vi "Authorization Read License File.vi"(8 "error in (no error)":errorcluster, 11 "Debug?":bool) -> (0 "error out":errorcluster, 3 "Authorization":T1)   [LabVIEW 2011]
uses:
  Authorization Data.ctl
  Authorization Global.vi
  <vilib>/xml/Load XML File.vi
  <vilib>/xml/Close Reference(Node).vi
  <vilib>/xml/NI_XML.lvlib
  Program Files/National Instruments/LabVIEW 2011/resource/objmgr/DOMUserDefRef.rc
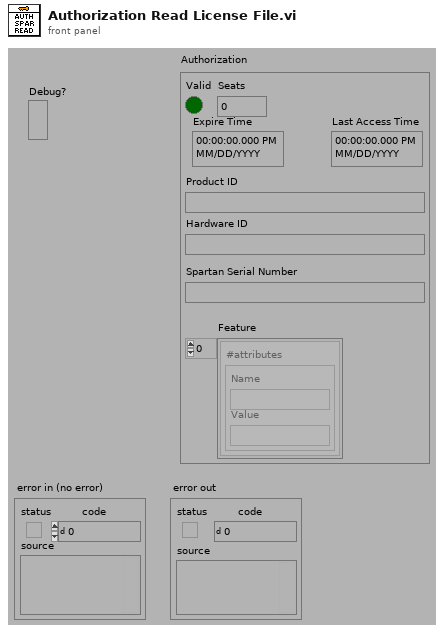
[diagram p1: front panel]
types:
  T1 = typedef "Authorization Data.ctl" = cluster{"Valid":bool, "Seats":i32, "Expire Time":timestamp, "Last Access Time":timestamp, "Product ID":string, "Hardware ID":string, "Spartan Serial Number":string, "Feature":cluster{"#attributes":cluster{"Name":string, "Value":string}}[]}
  T2 = enum32{"invalid app kind", "Development System", "Run Time System", "Student Edition", "Embedded LabVIEW", "Evaluation", "Custom"}
  T3 = cluster{"#attributes":cluster{"Name":string, "Value":string}}[]
  T4 = cluster{"#attributes":cluster{"Name":string, "Value":string}}
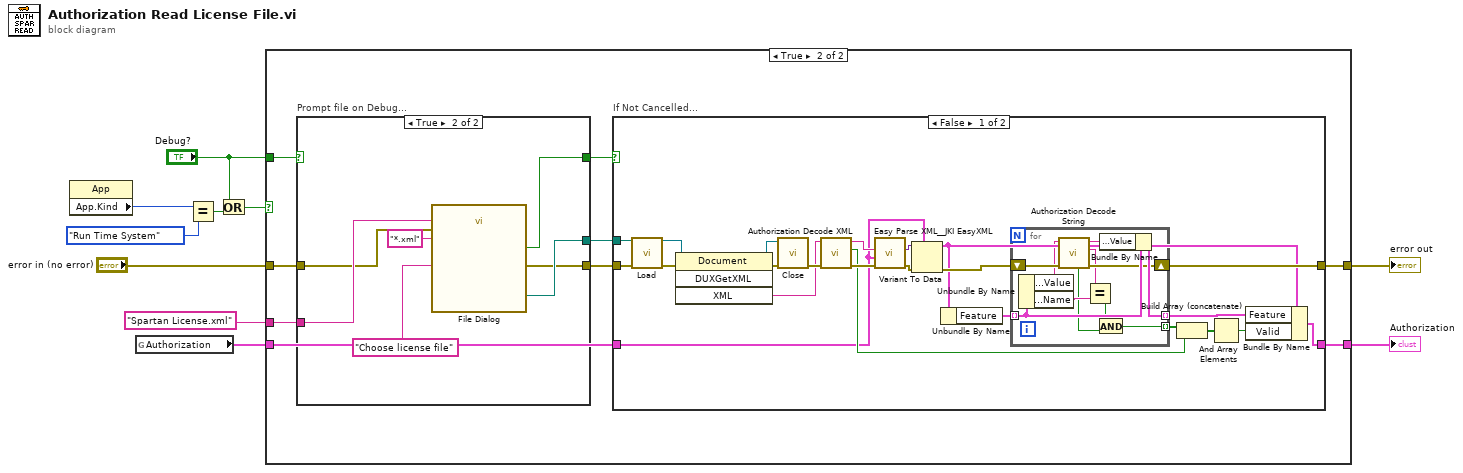
[diagram p0: block diagram]
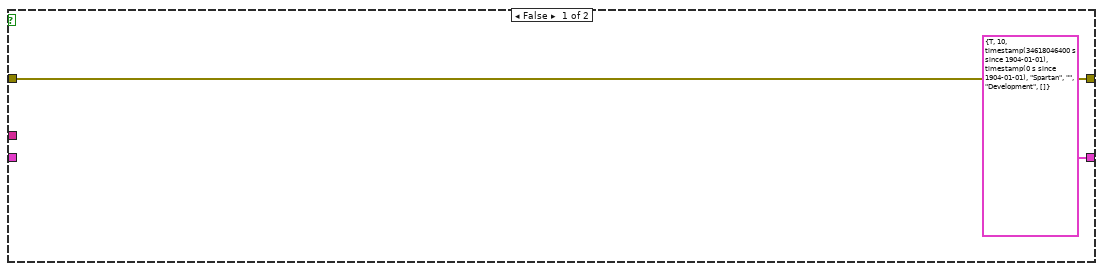
[diagram p2: hidden frame]
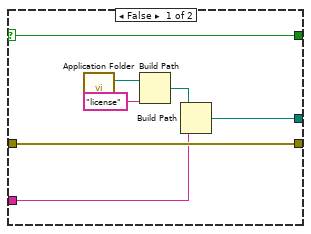
[diagram p4: hidden frame]
diagram:
  n1 = property class="App"() -> ("App.Kind"=w6:T2)  [unwired: 2 in, 2 out]
  n2 = global read "Authorization Global.vi" "Authorization"() -> (w1:T1)
  n3 = Equal?(x=w6, y=T2."Run Time System" ("t")) -> (x = y?=w4:bool)
  n4 = Or(x="Debug?", y=w4) -> (x .or. y?=w3:bool)
  n5 = case shown="True" w3 {
    tunnel: "error in (no error)" -> [w12 w16]
    tunnel: [w12 w21] -> w9
    tunnel: [T1 {"Valid"=TRUE, "Seats"=10, "Expire Time"=timestamp(34618046400 s since 1904-01-01), "Last Access Time"=timestamp(0 s since 1904-01-01), "Product ID"="Spartan", "Hardware ID"="", "Spartan Serial Number"="Development", "Feature"=[]} ("Authorization") w20] -> w8
    tunnel: "Spartan License.xml" ("default name") -> [_ w18]
    tunnel: "Debug?" -> [_ w17]
    tunnel: w1 -> [_ w13]
    frame False {
    }
    frame True {
      n6 = case "Prompt file on Debug..." shown="True" w17 {
        selector: w17 -> [w63 _]
        tunnel: [w58 w71] -> w19
        tunnel: w18 -> [w59 w68]
        tunnel: [w64 w66] -> w15
        tunnel: w16 -> [w64 w67]
        tunnel: [w63 w65] -> w14
        frame False {
          n7 = call "Application Folder.vi"() -> ("Application Folder"=w62:path)  [unwired: 3 in]
          n8 = Build Path(base path=w62, name or relative path="license" ("Relative Path (\"\" - Folder)")) -> (appended path=w60:path)
          n9 = Build Path(base path=w60, name or relative path=w59) -> (appended path=w58:path)
        }
        frame True {
          n10 = call "File Dialog"("prompt"="Choose license file", "default name"=w68, "error in"=w67, "pattern (all files)"="*.xml") -> ("selected path"=w71:path, "cancelled"=w65:bool, "error out"=w66:errorcluster)  [unwired: 8 in, 1 out]
        }
      }
      n11 = case "If Not Cancelled..." shown="False" w14 {
        tunnel: [w42 w57] -> w21
        tunnel: [w41 w56] -> w20
        tunnel: w19 -> [w40 _]
        tunnel: w15 -> [w39 w57]
        tunnel: w13 -> [w22 w56]
        frame False {
          n12 = call-poly <vilib>:"Load.vi"("path to XML document"=w40, "error in (no error)"=w39) -> ("DOM document out"=w44:refnum<k20>, "error out"=w43:errorcluster)  [unwired: 11 in, 1 out]
          n13 = invoke class="Document" method="DUXGetXML"(reference=w44, error in=w43) -> (reference out=w37:refnum<k20>, error out=w38:errorcluster, "XML"=w35:string)  [unwired: 2 in, 1 out]
          n14 = call-poly <vilib>:"Close.vi"("error in (no error)"=w38, "node"=w37) -> ("error out"=w36:errorcluster)  [unwired: 7 in]
          n15 = call "Authorization Decode XML.vi"("error in (no error)"=w36, "Encoded XML String"=w35) -> ("error out"=w32:errorcluster, "Valid"=w23:bool, "Decoded XML String"=w31:string)  [unwired: 7 in]
          n16 = call "Easy Parse XML__JKI EasyXML.vi"("error in (no error)"=w32, "LabVIEW Data (Type)"=w22, "XML String"=w31) -> ("error out"=w34:errorcluster, "LabVIEW Data"=w33:variant)  [unwired: 7 in]
          n17 = Variant To Data(error in=w34, type=w22, Variant=w33) -> (data=w28:T1, error out=w29:errorcluster)
          n18 = Unbundle By Name(w28) -> ("Feature"=w30:T3)
          n19 = for {
            tunnel: w30 -> [w55] mode=indexing
            tunnel: [w54] -> w27 mode=indexing
            shift-right: [w52] -> w42
            shift-left: w29 -> [w53]
            tunnel: [w45] -> w24 mode=indexing
            n20 = Unbundle By Name(w55) -> ("#attributes.Value"=w51:string, "#attributes.Name"=w50:string)
            n21 = call "Authorization Decode String.vi"("error in (no error)"=w53, "Encoded String"=w51) -> ("error out"=w52:errorcluster, "Property Name"=w49:string, "Decoded String"=w46:string, "Valid?"=w47:bool)  [unwired: 4 in, 2 out]
            n22 = Equal?(x=w49, y=w50) -> (x = y?=w48:bool)
            n23 = And(x=w48, y=w47) -> (x .and. y?=w45:bool)
            n24 = Bundle By Name(cluster=w55, "#attributes.Value"=w46) -> (w54:T4)
          }
          n25 = Build Array (concatenate)(w24, w23) -> (w26:bool[])
          n26 = And Array Elements(Boolean array=w26) -> (logical AND=w25:bool)
          n27 = Bundle By Name(cluster=w28, "Feature"=w27, "Valid"=w25) -> (w41:T1)
        }
        frame True {
        }
      }
    }
  }
  "error out" <- w9
  "Authorization" <- w8
